vi "Cmd_MoveToLimit.vi"(11 "Msg Data":variant) -> ()   [LabVIEW 2011]
uses:
  Main/Motors/MotorCmd_MoveToLimit.ctl
  Main/Motors/MotorAxisEnum.ctl
  PIAxisInfoGlobal.vi
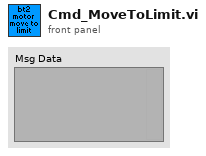
[diagram p1: front panel]
types:
  T1 = typedef "MotorCmd_MoveToLimit.ctl" = cluster{"Motor Axis":T2, "Limit switch":enum16{"Positive", "Negative"}}
  T2 = typedef "MotorAxisEnum.ctl" = enum16{"no axis", "magrot", "magpos", "px", "py", "pz", "camx", "camy"}
  T3 = typedef "GCS_Interface.ctl" = cluster{"MOV":refnum<vi>, "VEL":refnum<vi>, "VEL?":refnum<vi>, "POS?":refnum<vi>, "TMX?":refnum<vi>, "#7 (Ready?)":refnum<vi>, "FPL":refnum<vi>, "FNL":refnum<vi>}
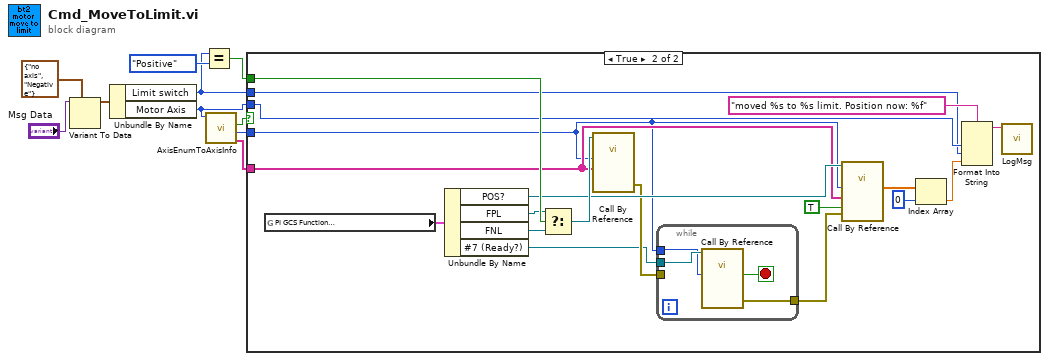
[diagram p0: block diagram]
diagram:
  n1 = Variant To Data(type=T1 {"Motor Axis"=enum."no axis", "Limit switch"=enum."Negative"} ("MotorCmd_MoveToLimit"), Variant="Msg Data") -> (data=w4:T1)  [unwired: 1 in, 1 out]
  n2 = Unbundle By Name(w4) -> ("Limit switch"=w1:enum16{"Positive", "Negative"}, "Motor Axis"=w9:T2)
  n3 = Equal?(x=w1, y=enum16{"Positive", "Negative"}."Positive") -> (x = y?=w6:bool)
  n4 = call "AxisEnumToAxisInfo.vi"("Motor Axis"=w9) -> ("Axis ID"=w8:string[], "System #"=w7:i32, "Valid axis?"=w5:bool)  [unwired: 6 in, 2 out]
  n5 = case shown="True" w5 {
    tunnel: w6 -> [_ w29]
    tunnel: w7 -> [_ w12]
    tunnel: w8 -> [_ w22]
    tunnel: w9 -> [_ w20]
    tunnel: w1 -> [_ w19]
    frame False {
    }
    frame True {
      n6 = global read "PIAxisInfoGlobal.vi" "PI GCS Function\nReferences"() -> (w28:T3)
      n7 = Unbundle By Name(w28) -> ("POS?"=w24:refnum<vi>, "FPL"=w27:refnum<vi>, "FNL"=w26:refnum<vi>, "#7 (Ready?)"=w13:refnum<vi>)
      n8 = Select(t=w27, s=w29, f=w26) -> (s? t:f=w25:refnum<vi>)
      n9 = call-by-ref "?"(reference=w25, "System no."=w12, "Affected axes"=w22) -> ("error out"=w14:errorcluster)  [unwired: 18 in, 2 out]
      n10 = while {
        tunnel: w14 -> [_]
        tunnel: w13 -> [w33]
        tunnel: w12 -> [w32]
        tunnel: [w30] -> w11
        stop <- w31 stop-if-true
        n11 = call-by-ref "?"(reference=w33, "System no."=w32) -> ("Ready?"=w31:bool, "error out"=w30:errorcluster)  [unwired: 17 in, 3 out]
      }
      n12 = call-by-ref "?"(reference=w24, "System no."=w12, "Axes to query"=w22, "Axis identifier?"=TRUE, "error in"=w11) -> ("Position"=w18:dbl[])  [unwired: 15 in, 3 out]
      n13 = Index Array(array=w18, index=0) -> (element=w16:dbl)
      n14 = Format Into String(format string="moved %s to %s limit. Position now: %f", w20, w19, w16) -> (resulting string=w15:string)  [unwired: 2 in, 1 out]
      n15 = call "LogMsg.vi"("msg"=w15) -> ()  [unwired: 11 in]
    }
  }
